vi "Create.vi"() -> (7 "HTTP Manager Identity out":refnum<class "HTTP Manager Identity.lvclass">)   [LabVIEW 2020, in "Volatus.lvlib" / "HTTP Manager Identity.lvclass"]
uses:
  HTTP Manager Identity.lvclass
  HTTP Manager Identity.lvclass/HTTP Manager Identity.ctl
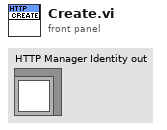
[diagram p1: front panel]
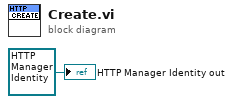
[diagram p0: block diagram]
diagram:
  "HTTP Manager Identity out" <- refnum<class "HTTP Manager Identity.lvclass"> refnum ("HTTP Manager Identity out")
